vi "Analog Input Voltages.vi"(8 "error in (no error)":errorcluster, 10 "Analog Input Voltages":waveform(dbl)[](array[waveform]), 11 "APG in":refnum<class "APG.lvclass">) -> (0 "error out":errorcluster, 3 "APG out":refnum<class "APG.lvclass">)   [LabVIEW 2021, in "APG.lvclass"]
uses:
  APG.lvclass
  APG.lvclass/APG.ctl
  <vilib>/Analysis/baseanly.llb/Mean (DBL).vi
  <vilib>/Analysis/NI_AALBase.lvlib
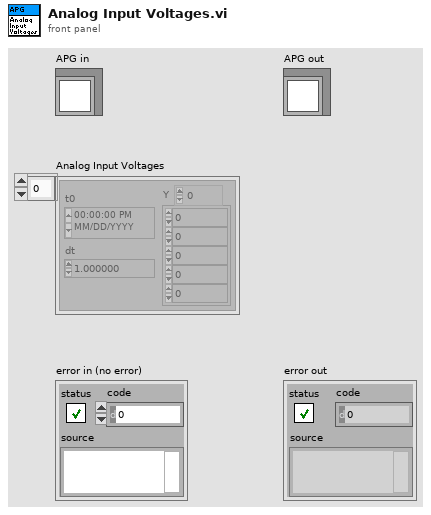
[diagram p1: front panel]
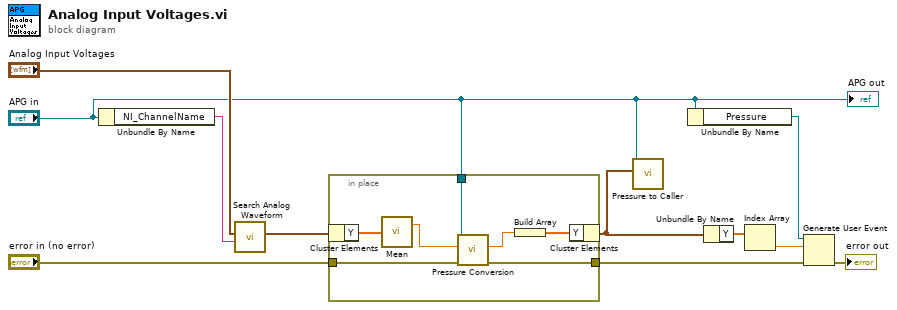
[diagram p0: block diagram]
diagram:
  n1 = Unbundle By Name("APG in") -> ("NI_ChannelName"=w9:string)
  n2 = call <vilib>:"Search Analog Waveform.vi"("NI_ChannelName"=w9, "Waveforms"="Analog Input Voltages") -> ("Waveform"=w5:waveform(dbl))  [unwired: 8 in, 1 out]
  n3 = in-place {
    in-place-border: [w18] -> w10
    in-place-border: "error in (no error)" -> [w16]
    in-place-border: "APG in" -> [w15]
    n4 = in-place-cluster #1(w5) -> ("Y"=w14:dbl[])
    n5 = call-poly <vilib>:"Mean.vi"("X"=w14) -> ("mean"=w17:dbl)  [unwired: 1 out]
    n6 = call "Pressure Conversion.vi"("error in (no error)"=w16, "Voltage"=w17, "APG in"=w15) -> ("error out"=w18:errorcluster, "Pressure"=w13:dbl)  [unwired: 7 in]
    n7 = Build Array(w13) -> (w12:dbl[])
    n8 = in-place-cluster #1("Y"=w12) -> (w4:waveform(dbl))
  }
  n9 = call-dynamic "Pressure to Caller.vi"("Analog Input Waveform"=w4, "APG in"="APG in") -> ()  [unwired: 9 in, 1 out]
  n10 = Unbundle By Name("APG in") -> ("Pressure"=w11:refnum<user-event>)
  n11 = Unbundle By Name(w4) -> ("Y"=w2:dbl[])
  n12 = Index Array(array=w2) -> (element=w1:dbl)  [unwired: 1 in]
  n13 = Generate User Event(user event=w11, event data cluster=w1, error in=w10) -> (error out=→"error out":errorcluster)  [unwired: 1 in, 1 out]
  "APG out" <- "APG in"
